vi "GUI_BELLA_ESP.vi"() -> ()   [LabVIEW 2013]
uses:
  Shared/GUI_Template/GUI_master/tcp_new_data_event.ctl
  Shared/GUI_Template/GUI_master/tcp new data cluster.ctl
panel:
  in  "stop":bool
  in  "Status.Axis 2::3":T1(ring) caption="Status"
  in  "Home.Axis 2::3":dbl=0.5 caption="Home" min=0.0 max=6.0 format="%_4f"
  in  "Power.Axis 2::3":enum16{"on", "off"}(ring) caption="Power"
  in  "Position.Axis 2::3":dbl=0.5 caption="Position" min=-12.0 max=10.0 format="%_4f"
  in  "Status.Axis 3::3":T1(ring) caption="Status"
  in  "Home.Axis 3::3":dbl=0.5 caption="Home" min=0.0 max=6.0 format="%_4f"
  in  "Power.Axis 3::3":enum16{"on", "off"}(ring) caption="Power"
  in  "Position.Axis 3::3":dbl=0.5 caption="Position" min=-12.0 max=12.0 format="%_4f"
  in  "Status.Axis 1::3":T1(ring) caption="Status"
  in  "Home.Axis 1::3":dbl=0.5 caption="Home" min=0.0 max=6.0 format="%_4f"
  in  "Power.Axis 1::3":enum16{"on", "off"}(ring) caption="Power"
  in  "Position.Axis 1::3":dbl=0.5 caption="Position" min=-10.0 max=10.0 format="%_4f"
  in  "Status.Axis 3::2":T1(ring) caption="Status"
  in  "Home.Axis 3::2":dbl=0.5 caption="Home" min=0.0 max=6.0 format="%_4f"
  in  "Power.Axis 3::2":enum16{"on", "off"}(ring) caption="Power"
  in  "Position.Axis 3::2":dbl=0.5 caption="Position" min=-10.0 max=10.0 format="%_4f"
  in  "Status.Axis 2::2":T1(ring) caption="Status"
  in  "Home.Axis 2::2":dbl=0.5 caption="Home" min=0.0 max=6.0 format="%_4f"
  in  "Power.Axis 2::2":enum16{"on", "off"}(ring) caption="Power"
  in  "Position.Axis 2::2":dbl=0.5 caption="Position" min=-6.0 max=3.0 format="%_4f"
  in  "Status.Axis 1::2":T1(ring) caption="Status"
  in  "Home.Axis 1::2":dbl=0.5 caption="Home" min=0.0 max=6.0 format="%_4f"
  in  "Power.Axis 1::2":enum16{"on", "off"}(ring) caption="Power"
  in  "Position.Axis 1::2":dbl=0.5 caption="Position" min=-8.0 max=3.0 format="%_4f"
  in  "Status.Axis 2::1":T1(ring) caption="Status"
  in  "Home.Axis 2::1":dbl=0.5 caption="Home" min=0.0 max=6.0 format="%_4f"
  in  "Power.Axis 2::1":enum16{"on", "off"}(ring) caption="Power"
  in  "Position.Axis 2::1":dbl=0.5 caption="Position" min=-3.0 max=3.0 format="%_4f"
  in  "Status.Axis 1::1":T1(ring) caption="Status"
  in  "Home.Axis 1::1":dbl=0.5 caption="Home" min=0.0 max=6.0 format="%_4f"
  in  "Power.Axis 1::1":enum16{"on", "off"}(ring) caption="Power"
  in  "Position.Axis 1::1":dbl=0.5 caption="Position" min=-10.0 max=10.0 format="%_4f"
  out "error IO 2":errorcluster
  out "tcp data event":T2
  in  "GUIdevice 3":string="BELLA_ESP_2"
  in  "GUIdevice 1":string="BELLA_ESP_M1"
  in  "GUIdevice 2":string="BellaESP"
  in  "insert tag":bool=TRUE
  # "Horizontal"
  # "BELLA PW ESP301"
  # "M5 AXIS 1"
  # "Horizontal"
  # "M5 AXIS 2"
  # "Vertical"
  # "M4 AXIS 2"
  # "Horizontal"
  # "M4 AXIS 1"
  # "Vertical"
  # "M2 AXIS 2"
  # "Horizontal"
  # "M2 AXIS 1"
  # "Vertical"
  # "M1 AXIS 2"
  # "Horizontal"
  # "M1 AXIS 1"
  # "Vertical"
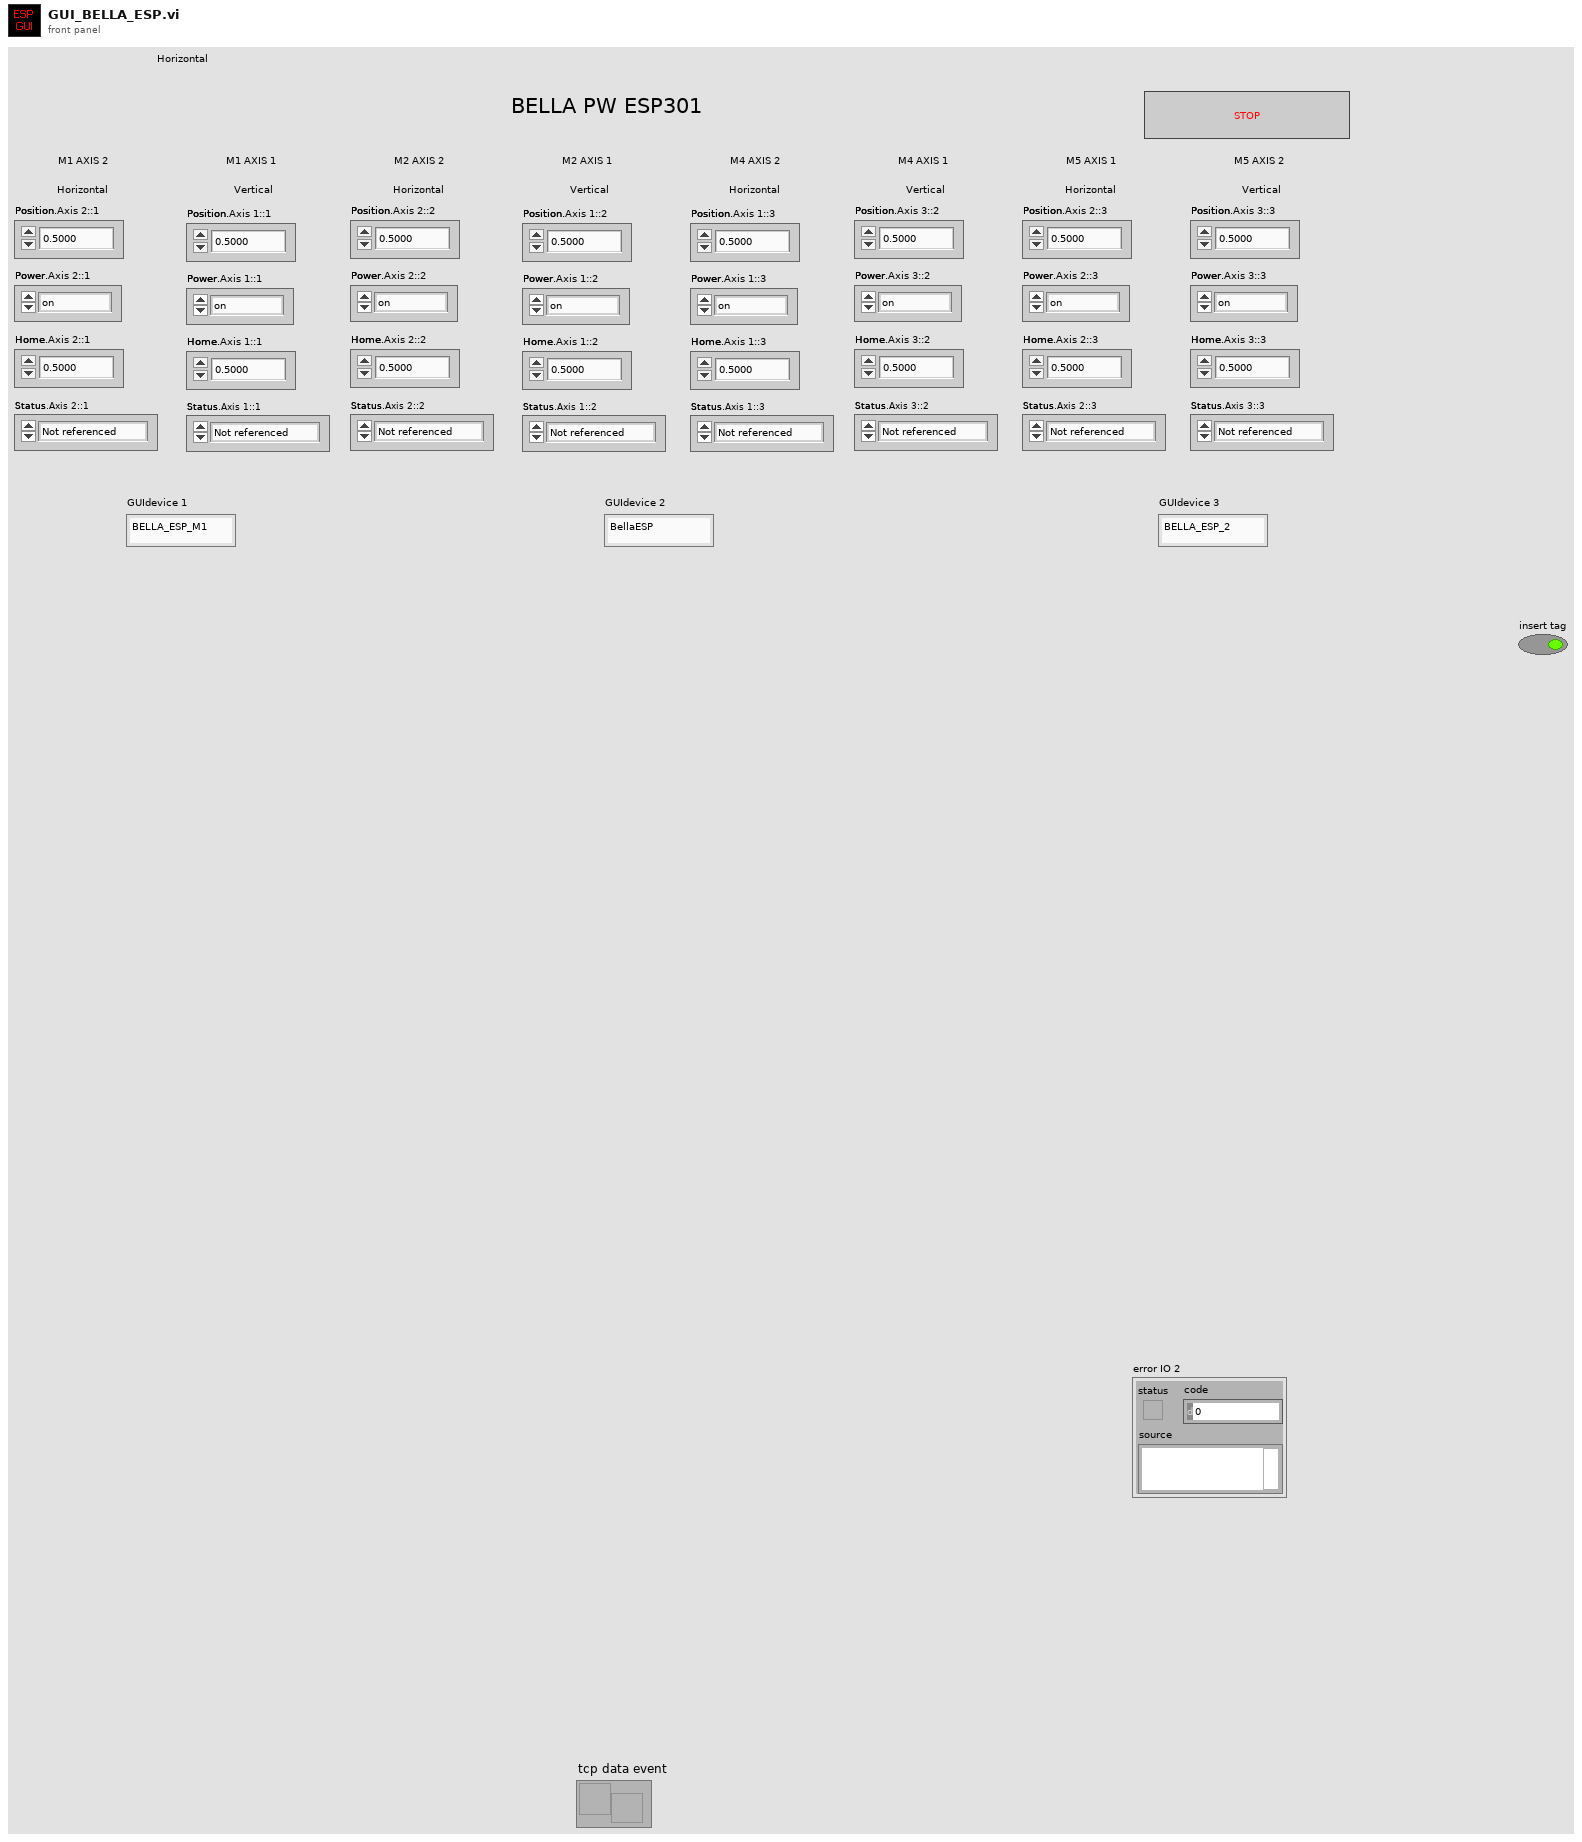
[diagram p1: front panel]
types:
  T1 = enum16{"Not referenced", "Homing", "Moving", "Ready"}
  T2 = typedef "tcp_new_data_event.ctl" = refnum<user-event>
  T3 = typedef "tcp new data cluster.ctl" = cluster{"EventEnum":enum16{"new data", "connection status update"}, "Device name":string}
  T4 = enum32{"Invalid", "Standard", "Closed", "Hidden", "Minimized", "Maximized"}
  T5 = enum32{"invalid app kind", "Development System", "Run Time System", "Student Edition", "Embedded LabVIEW", "Evaluation", "Custom"}
  T6 = cluster{"Core":cluster{"Current VI Reference":refnum<vi>, "Close Panel on Exit?":bool}, "Your Boolean data":bool, "Your string data":string}
  T7 = cluster{"Current VI Reference":refnum<vi>, "Close Panel on Exit?":bool}
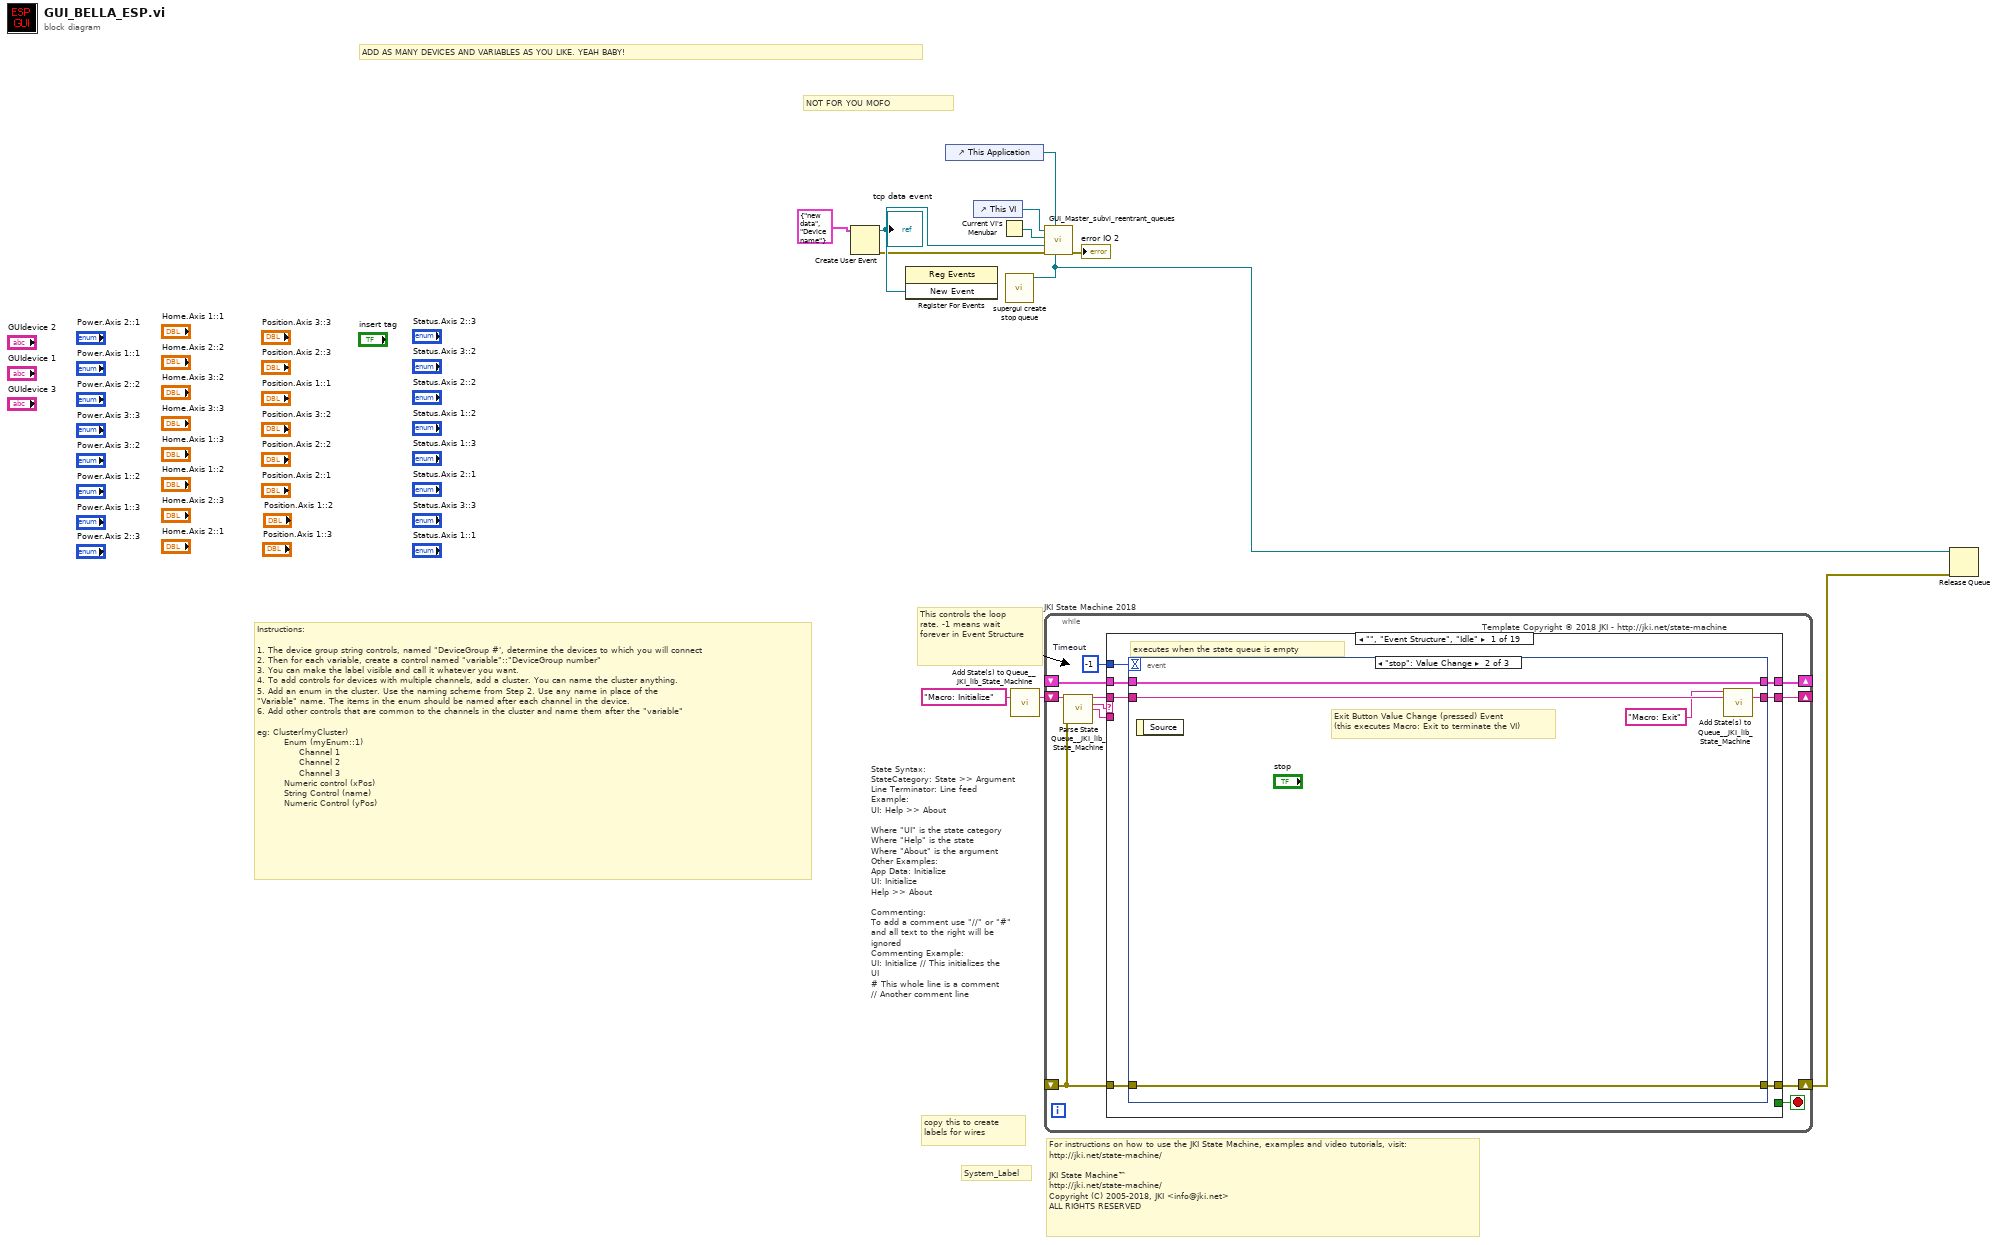
[diagram p0: block diagram]
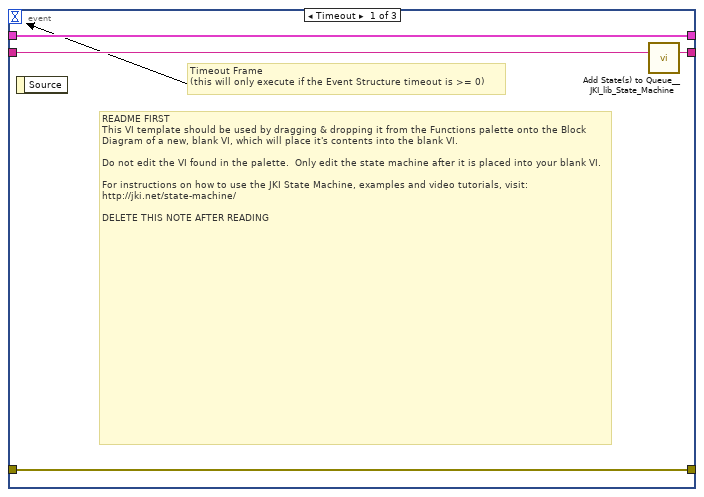
[diagram p2: hidden frame]
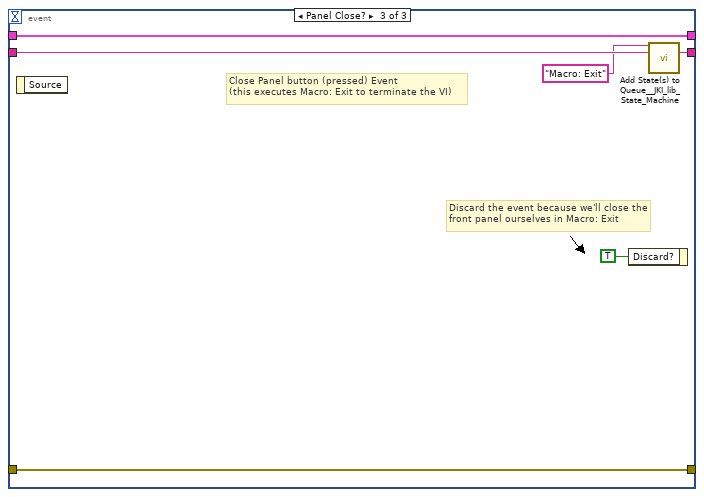
[diagram p3: hidden frame]
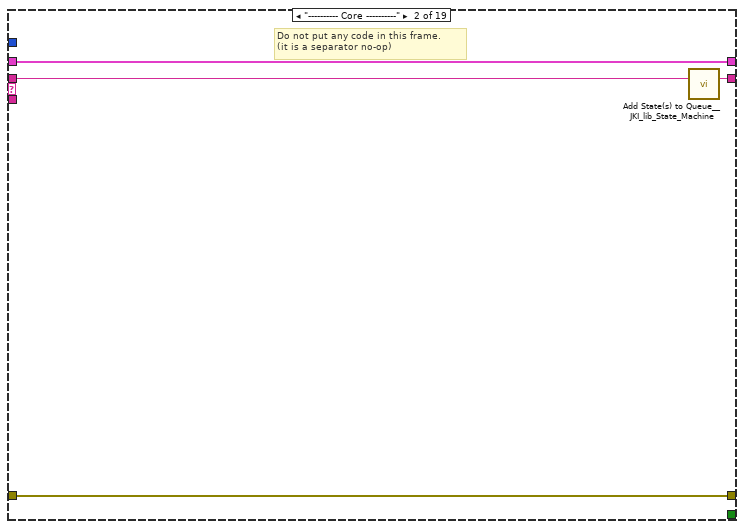
[diagram p4: hidden frame]
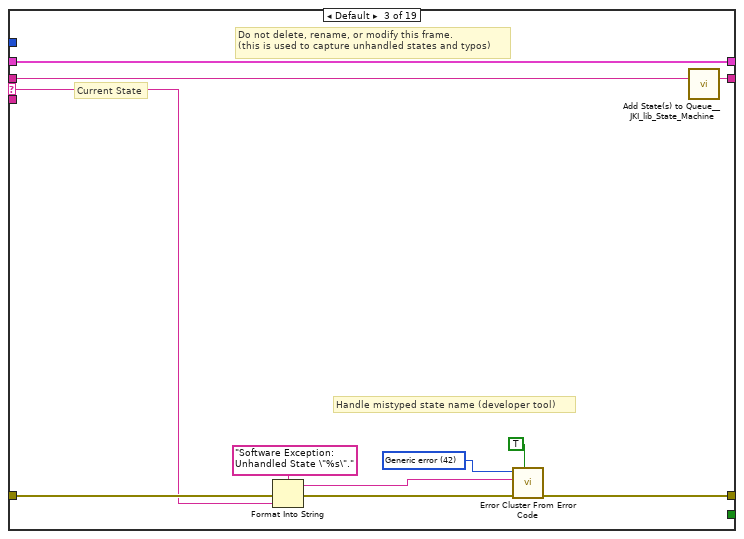
[diagram p5: hidden frame]
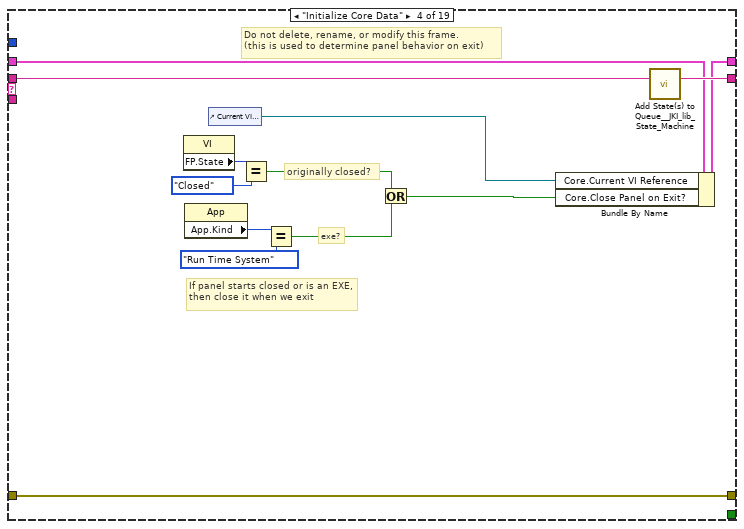
[diagram p6: hidden frame]
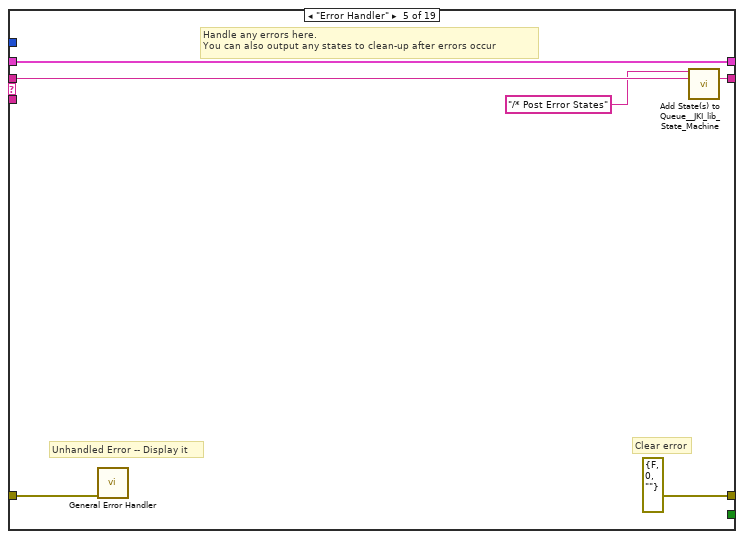
[diagram p7: hidden frame]
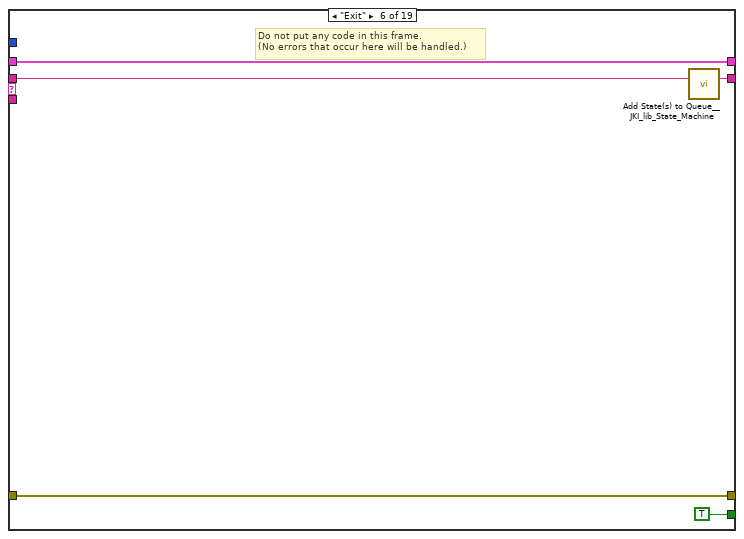
[diagram p8: hidden frame]
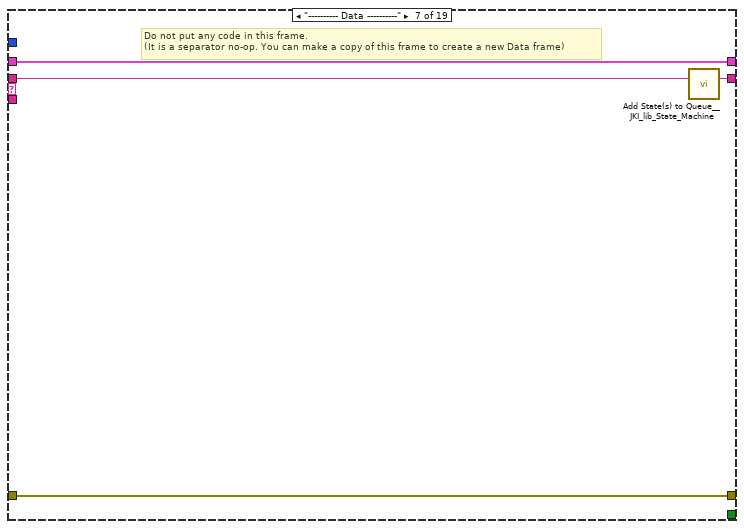
[diagram p9: hidden frame]
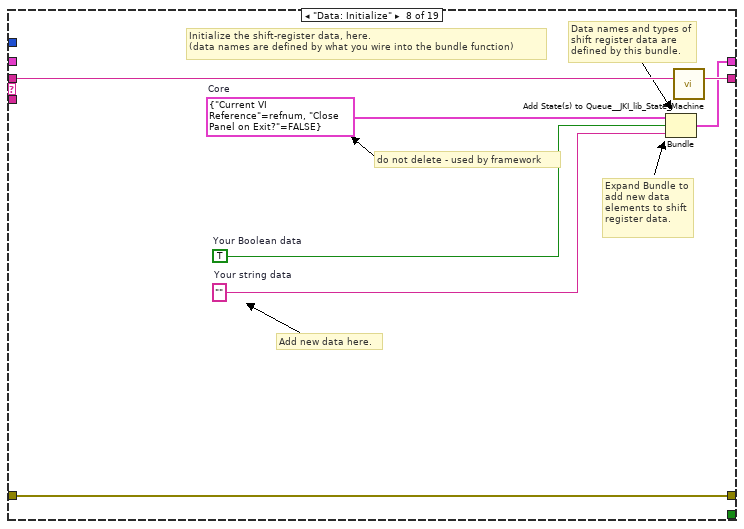
[diagram p10: hidden frame]
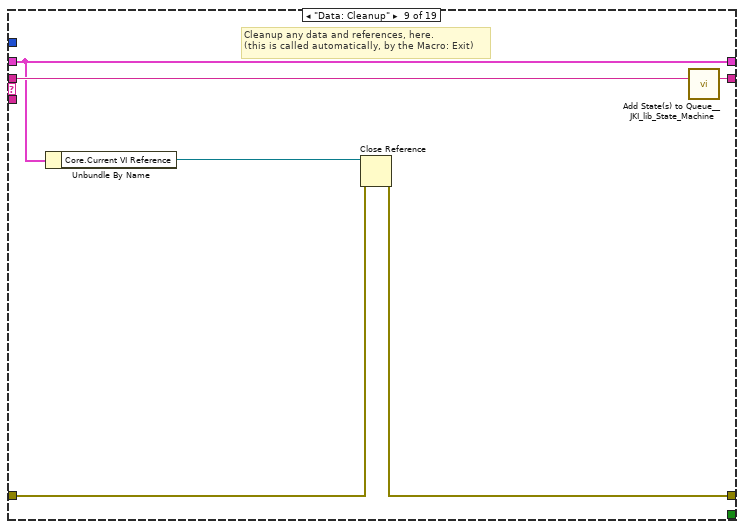
[diagram p11: hidden frame]
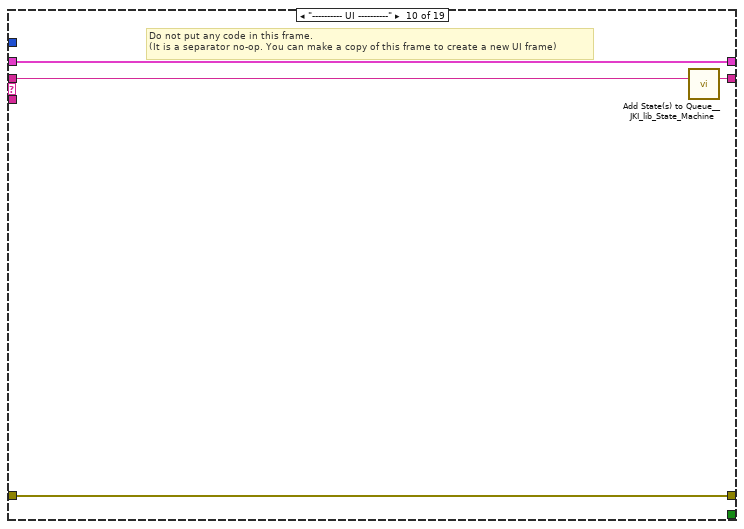
[diagram p12: hidden frame]
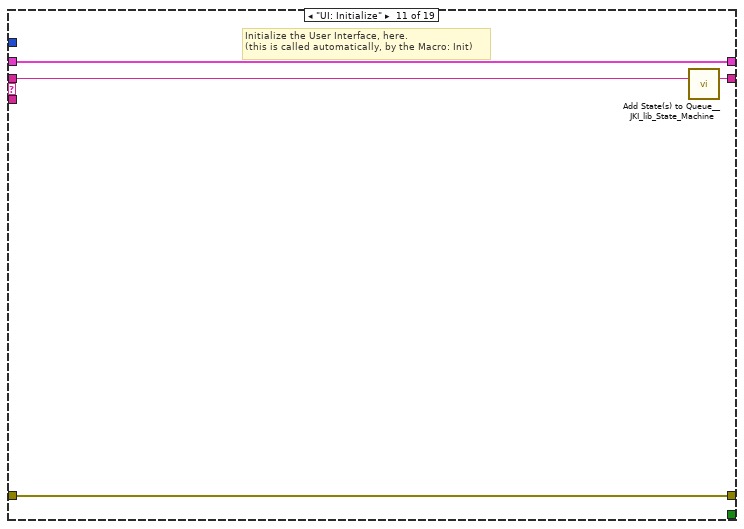
[diagram p13: hidden frame]
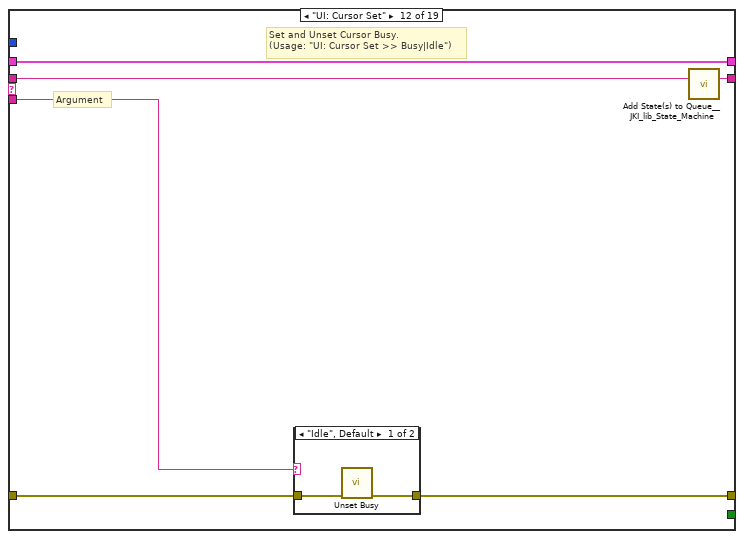
[diagram p14: hidden frame]
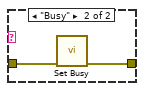
[diagram p15: hidden frame]
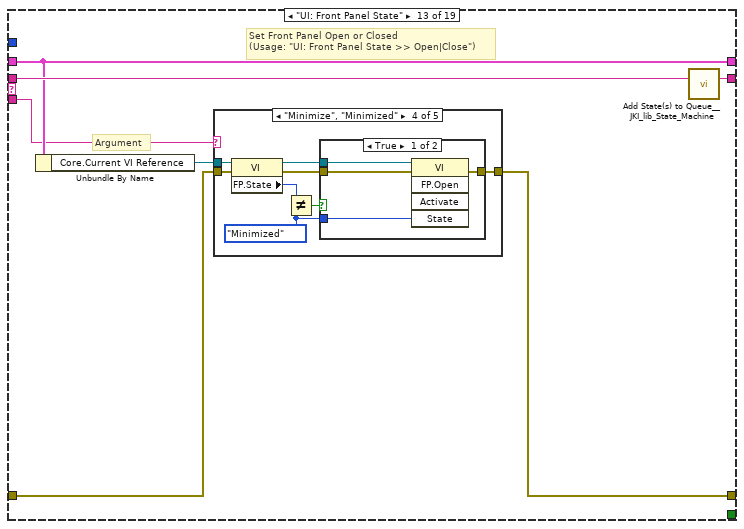
[diagram p16: hidden frame]
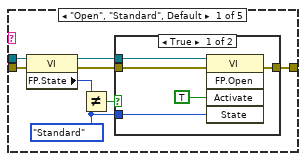
[diagram p17: hidden frame]
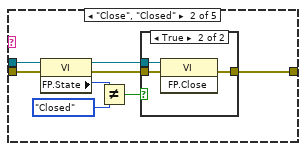
[diagram p19: hidden frame]
diagram:
  # "For instructions on how to use the JKI State Machine, examples and video tutorials, visit:\nhttp://jki.net/state-machine/\n\nJKI State Machine™\nhttp://jki.net/state-machine/\nCopyright (C) 2005-2018, JKI <info@jki.net>\nALL RIGHTS RESERVED"
  # "State Syntax:\nStateCategory: State >> Argument\nLine Terminator: Line feed\nExample:\nUI: Help >> About\n\nWhere \"UI\" is the state category\nWhere \"Help\" is the state\nWhere \"About\" is the argument\nOther Examples:\nApp Data: Initialize\nUI: Initialize\nHelp >> About\n\nCommenting:\nTo add a comment use \"//\" or \"#\" and all text to the right will be ignored\nCommenting Example:\nUI: Initialize // This initializes the UI\n# This whole line is a comment\n// Another comment line"
  # "copy this to create labels for wires"
  # "This controls the loop rate. -1 means wait forever in Event Structure"
  # "System_Label"
  # "NOT FOR YOU MOFO"
  # "Instructions:\n\n1. The device group string controls, named \"DeviceGroup #', determine the devices to which you will connect\n2. Then for each variable, create a control named \"variable\"::\"DeviceGroup number\"\n3. You can make the label visible and call it whatever you want.\n4. To add controls for devices with multiple channels, add a cluster. You can name the cluster anything.\n5. Add an enum in the cluster. Use the naming scheme from Step 2. Use any name in place of the \n\"Variable\" name. The items in the enum should be named after each channel in the device. \n6. Add other controls that are common to the channels in the cluster and name them after the \"variable\"\n\neg: Cluster(myCluster)\n         Enum (myEnum::1)\n              Channel 1 \n              Channel 2\n              Channel 3\n         Numeric control (xPos)\n         String Control (name)\n         Numeric Control (yPos)"
  # "ADD AS MANY DEVICES AND VARIABLES AS YOU LIKE. YEAH BABY!"
  n1 = Create User Event(user event datatype=T3 {"EventEnum"=enum."new data", "Device name"="Device name"} ("New Event")) -> (user event=w10:refnum<user-event>, error out=w9:errorcluster)  [unwired: 1 in]
  "tcp data event" <- w10
  n2 = register-events(w10) -> ()  [unwired: 2 in, 2 out]
  n3 = control-ref of="This Application"() -> (w11:refnum<vi>)
  n4 = control-ref of="This VI"() -> (w6:refnum<vi>)
  n5 = Current VI's Menubar() -> (w7:refnum<k9>)
  n6 = call "supergui create stop queue.vi"() -> ("STOP Queue out"=w4:refnum<queue>)  [unwired: 11 in]
  n7 = call <vilib>:"Add State(s) to Queue__JKI_lib_State_Machine.vi"("State(s) in (\"\")"="Macro: Initialize") -> ("States Out"=w3:string)  [unwired: 14 in]
  n8 = call "GUI_Master_subvi_reentrant_queues.vi"("STOP Queue in"=w4, "This Application"=w11, "error in (no error)"=w9, "tcp data event"=w10, "Caller menu reference"=w7, "Caller VI ref"=w6) -> ("error out"=→"error IO 2":errorcluster)  [unwired: 5 in]
  n9 = while "JKI State Machine 2018" {
    shift-right: [w15] -> _
    shift-left: _ -> [w14]
    shift-right: [w18] -> w1
    shift-left: _ -> [w12]
    shift-right: [w17] -> _
    shift-left: w3 -> [w19]
    stop <- w16 stop-if-true
    w13 = -1  # Timeout
    # "Template Copyright © 2018 JKI - http://jki.net/state-machine"
    n10 = call <vilib>:"Parse State Queue__JKI_lib_State_Machine.vi"("State Queue"=w19, "Error In (no error)"=w12) -> ("Remaining States"=w21:string, "Current State"=w22:string, "Arguments"=w20:string)  [unwired: 11 in]
    n11 = case shown="\"\", \"Event Structure\", \"Idle\"" w22 {
      selector: w22 -> [_ _ w49 _ _ _ _ _ _ _ _ _ _ _ _ _ _ _ _]
      tunnel: w21 -> [w29 w48 w53 w72 w78 w83 w87 w94 w100 w104 w108 w114 w125 w194 w199 w209 w213 w217 w221]
      tunnel: w20 -> [_ _ _ _ _ _ _ _ _ _ _ w109 w119 _ _ _ _ _ _]
      tunnel: w14 -> [w27 w45 w51 w65 w75 w81 w84 _ w95 w101 w106 w112 w121 w191 w196 w206 w210 w214 w218]
      tunnel: [w26 w46 w55 w69 errorcluster {"status"=FALSE, "code"=0, "source"=""} ("error out") w80 w85 w91 w96 w102 w105 w110 w122 w192 w197 w207 w211 w215 w219] -> w18
      tunnel: w12 -> [w25 w46 w54 w69 w74 w80 w85 w91 w97 w102 w105 w111 w123 w192 w197 w207 w211 w215 w219]
      tunnel: [w28 w47 w52 w71 w77 w82 w86 w93 w99 w103 w107 w113 w124 w193 w198 w208 w212 w216 w220] -> w17
      tunnel: [_ _ _ _ _ TRUE _ _ _ _ _ _ _ _ _ _ _ _ _] -> w16
      tunnel: [w24 w45 w51 w70 w75 w81 w84 w92 w95 w101 w106 w112 w121 w191 w196 w206 w210 w214 w218] -> w15
      tunnel: w13 -> [w23 _ _ _ _ _ _ _ _ _ _ _ _ _ _ _ _ _ _]
      frame "", "Event Structure", "Idle" {
        # "executes when the state queue is empty"
        n12 = event shown="[1] \"stop\": Value Change" {
          selector: _ -> [_ _ _]
          dyn-events: _ -> [_ _ _]
          timeout: w23 -> [_ _ _]
          tunnel: w29 -> [w33 w38 w44]
          tunnel: [w32 w37 w43] -> w28
          tunnel: w27 -> [w30 w35 w41]
          tunnel: [w31 w36 w42] -> w26
          tunnel: w25 -> [w31 w36 w42]
          tunnel: [w30 w35 w41] -> w24
          event Timeout {
            # "README FIRST\nThis VI template should be used by dragging & dropping it from the Functions palette onto the Block Diagram of a new, blank VI, which will place it's contents into the blank VI.\n\nDo not edit the VI found in the palette.  Only edit the state machine after it is placed into your blank VI.\n\nFor instructions on how to use the JKI State Machine, examples and video tutorials, visit:\nhttp://jki.net/state-machine/\n\nDELETE THIS NOTE AFTER READING"
            # "Timeout Frame\n(this will only execute if the Event Structure timeout is >= 0)"
            n13 = event-data() -> ()  [unwired: 1 in, 1 out]
            n14 = call <vilib>:"Add State(s) to Queue__JKI_lib_State_Machine.vi"("State(s) in (\"\")"=w33) -> ("States Out"=w32:string)  [unwired: 14 in]
          }
          event "stop": Value Change {
            # "Exit Button Value Change (pressed) Event\n(this executes Macro: Exit to terminate the VI)"
            n15 = event-data() -> ()  [unwired: 1 in, 1 out]
            n16 = call <vilib>:"Add State(s) to Queue__JKI_lib_State_Machine.vi"("State(s) in Front (\"\")"="Macro: Exit", "State(s) in (\"\")"=w38) -> ("States Out"=w37:string)  [unwired: 13 in]
          }
          event Panel Close? {
            # "Discard the event because we'll close the front panel ourselves in Macro: Exit"
            # "Close Panel button (pressed) Event\n(this executes Macro: Exit to terminate the VI)"
            n17 = event-data() -> ()  [unwired: 1 in, 1 out]
            n18 = event-data("Discard?"=TRUE) -> ()  [unwired: 1 in, 1 out]
            n19 = call <vilib>:"Add State(s) to Queue__JKI_lib_State_Machine.vi"("State(s) in Front (\"\")"="Macro: Exit", "State(s) in (\"\")"=w44) -> ("States Out"=w43:string)  [unwired: 13 in]
          }
        }
      }
      frame "---------- Core ----------" {
        # "Do not put any code in this frame.\n(it is a separator no-op)"
        n20 = call <vilib>:"Add State(s) to Queue__JKI_lib_State_Machine.vi"("State(s) in (\"\")"=w48) -> ("States Out"=w47:string)  [unwired: 14 in]
      }
      frame Default {
        w58 = 42 items=["No error", "Argument error", "Memory is full", "Out of zone", "End of file", "File already open", "Generic file I/O error", "File not found", "File permission error", "Disk is full", "Duplicate path", "Too many files open", "System feature not enabled", "Resource file not found", "Cannot add resource", "Resource not found", "Image not found", "Image memory error", "Pen does not exist", "Config type invalid", "Config token not found", "Config parse error", "Config memory error", "Bad external code format", "Bad external code offset", "External code not present", "Null window", "Destroy window error", "Null menu", "Print aborted", "Bad print record", "Print driver error", "Windows error during printing", "Memory error during printing", "Print dialog error", "Generic print error", "Invalid device refnum", "Device not found", "Device parameter error", "Device unit error", "Cannot open device", "Device call aborted", "Generic error", "Cancelled by user", "Object ID too low", "Object ID too high", "Object not in heap", "Unknown heap", "Unknown object (invalid DefProc)", "Unknown object (DefProc not in table)", "Message out of range", "Invalid (null) method", "Unknown message", "Manager call not supported", "Bad address", "Network operation in progress", "Network operation timed out", "Connection is busy", "Network attribute not supported", "Network error", "Address in use", "System out of memory", "Connection aborted", "Connection refused", "Not connected", "Already connected", "Connection closed", "Initialization error (interapplication manager)", "Bad occurrence", "Wait on unbound occurrence handler", "Occurrence queue overflow", "Datalog type conflict", "Unused", "Unrecognized type (interapplication manager)", "Memory corrupt", "Failed to make temporary DLL", "Old CIN version", "Drag socket not found", "Failed to load drop-object", "Failed to register OLE object", "Failed to release OLE object", "Format specifier type mismatch", "Unknown format specifier", "Too few format specifiers", "Too many format specifiers", "Scan failed", "Newer CIN version", "Error converting to variant", "Runtime menu error", "Password tampered", "Variant attribute not found", "Incompatible variant data type", "Event data is not available", "Event Store is not present", "Occurrence is not found", "Event Queue is not created", "Event info is not available", "Refnum passed is NULL", "Error retrieving Class GUID", "Error retrieving CoClass GUID", "Error retrieving TypeLib GUID.", "Bad built application magic bytes.", "Specific driver is different from the specific driver associated with the Logical Name.", "There is no session opened to the class driver.", "Max Error", "MAX - Error with config objects", "MAX - Error loading configuration", "MAX - Group not supported"]
        # "Current State"
        # "Do not delete, rename, or modify this frame.\n(this is used to capture unhandled states and typos)"
        # "Handle mistyped state name (developer tool)"
        n21 = Format Into String(format string="Software Exception: Unhandled State \"%s\"." ("message"), error in=w54, w49) -> (resulting string=w57:string, error out=w56:errorcluster)  [unwired: 1 in]
        n22 = call <vilib>:"Error Cluster From Error Code.vi"("show call chain? (False)"=TRUE, "error in (no error)"=w56, "error message (\"\")"=w57, "error code (0)"=w58) -> ("error out"=w55:errorcluster)  [unwired: 5 in]
        n23 = call <vilib>:"Add State(s) to Queue__JKI_lib_State_Machine.vi"("State(s) in (\"\")"=w53) -> ("States Out"=w52:string)  [unwired: 14 in]
      }
      frame "Initialize Core Data" {
        # "Do not delete, rename, or modify this frame.\n(this is used to determine panel behavior on exit)"
        # "originally closed?"
        # "exe?"
        # "If panel starts closed or is an EXE, then close it when we exit"
        n24 = property class="VI"() -> ("FP.State"=w62:T4)  [unwired: 2 in, 2 out]
        n25 = property class="App"() -> ("App.Kind"=w68:T5)  [unwired: 2 in, 2 out]
        n26 = control-ref of="Current VI Reference"() -> (w63:refnum<vi>)
        n27 = Equal?(x=w62, y=T4."Closed" ("Front Panel Window:State")) -> (x = y?=w60:bool)
        n28 = Equal?(x=w68, y=T5."Run Time System" ("Application:Kind")) -> (x = y?=w66:bool)
        n29 = Or(x=w60, y=w66) -> (x .or. y?=w64:bool)
        n30 = Bundle By Name(cluster=w65, "Core.Current VI Reference"=w63, "Core.Close Panel on Exit?"=w64) -> (w70:T6)
        n31 = call <vilib>:"Add State(s) to Queue__JKI_lib_State_Machine.vi"("State(s) in (\"\")"=w72) -> ("States Out"=w71:string)  [unwired: 14 in]
      }
      frame "Error Handler" {
        # "Unhandled Error -- Display it"
        # "Handle any errors here.\nYou can also output any states to clean-up after errors occur"
        # "Clear error"
        n32 = call <vilib>:"General Error Handler.vi"("error in (no error)"=w74) -> ()  [unwired: 10 in, 5 out]
        n33 = call <vilib>:"Add State(s) to Queue__JKI_lib_State_Machine.vi"("State(s) in Front (\"\")"="/* Post Error States", "State(s) in (\"\")"=w78) -> ("States Out"=w77:string)  [unwired: 13 in]
      }
      frame "Exit" {
        # "Do not put any code in this frame.\n(No errors that occur here will be handled.)"
        n34 = call <vilib>:"Add State(s) to Queue__JKI_lib_State_Machine.vi"("State(s) in (\"\")"=w83) -> ("States Out"=w82:string)  [unwired: 14 in]
      }
      frame "---------- Data ----------" {
        # "Do not put any code in this frame.\n(It is a separator no-op. You can make a copy of this frame to create a new Data frame)"
        n35 = call <vilib>:"Add State(s) to Queue__JKI_lib_State_Machine.vi"("State(s) in (\"\")"=w87) -> ("States Out"=w86:string)  [unwired: 14 in]
      }
      frame "Data: Initialize" {
        w88 = T7 {"Current VI Reference"=refnum, "Close Panel on Exit?"=FALSE}  # Core
        w90 = TRUE  # Your Boolean data
        w89 = ""  # Your string data
        # "do not delete - used by framework"
        # "Expand Bundle to add new data elements to shift register data."
        # "Add new data here."
        # "Data names and types of shift register data are defined by this bundle."
        # "Initialize the shift-register data, here.\n(data names are defined by what you wire into the bundle function)"
        n36 = Bundle("Core"=w88, "Your Boolean data"=w90, "Your string data"=w89) -> (w92:T6)  [unwired: 1 in]
        n37 = call <vilib>:"Add State(s) to Queue__JKI_lib_State_Machine.vi"("State(s) in (\"\")"=w94) -> ("States Out"=w93:string)  [unwired: 14 in]
      }
      frame "Data: Cleanup" {
        # "Cleanup any data and references, here.\n(this is called automatically, by the Macro: Exit)"
        n38 = Unbundle By Name(w95) -> ("Core.Current VI Reference"=w98:refnum<vi>)
        n39 = Close Reference(reference=w98, error in (no error)=w97) -> (error out=w96:errorcluster)
        n40 = call <vilib>:"Add State(s) to Queue__JKI_lib_State_Machine.vi"("State(s) in (\"\")"=w100) -> ("States Out"=w99:string)  [unwired: 14 in]
      }
      frame "---------- UI ----------" {
        # "Do not put any code in this frame.\n(It is a separator no-op. You can make a copy of this frame to create a new UI frame)"
        n41 = call <vilib>:"Add State(s) to Queue__JKI_lib_State_Machine.vi"("State(s) in (\"\")"=w104) -> ("States Out"=w103:string)  [unwired: 14 in]
      }
      frame "UI: Initialize" {
        # "Initialize the User Interface, here.\n(this is called automatically, by the Macro: Init)"
        n42 = call <vilib>:"Add State(s) to Queue__JKI_lib_State_Machine.vi"("State(s) in (\"\")"=w108) -> ("States Out"=w107:string)  [unwired: 14 in]
      }
      frame "UI: Cursor Set" {
        # "Argument"
        # "Set and Unset Cursor Busy.\n(Usage: \"UI: Cursor Set >> Busy|Idle\")"
        n43 = case shown="\"Idle\", Default" w109 {
          tunnel: w111 -> [w116 w118]
          tunnel: [w115 w117] -> w110
          frame "Idle", Default {
            n44 = call <vilib>:"Unset Busy.vi"("error in (no error)"=w116) -> ("error out"=w115:errorcluster)  [unwired: 10 in]
          }
          frame "Busy" {
            n45 = call <vilib>:"Set Busy.vi"("error in (no error)"=w118) -> ("error out"=w117:errorcluster)  [unwired: 9 in, 1 out]
          }
        }
        n46 = call <vilib>:"Add State(s) to Queue__JKI_lib_State_Machine.vi"("State(s) in (\"\")"=w114) -> ("States Out"=w113:string)  [unwired: 14 in]
      }
      frame "UI: Front Panel State" {
        # "Argument"
        # "Set Front Panel Open or Closed\n(Usage: \"UI: Front Panel State >> Open|Close\")"
        n47 = Unbundle By Name(w121) -> ("Core.Current VI Reference"=w120:refnum<vi>)
        n48 = case shown="\"Minimize\", \"Minimized\"" w119 {
          tunnel: w123 -> [w131 w146 w157 w170 w183]
          tunnel: [w133 w147 w159 w172 w185] -> w122
          tunnel: w120 -> [w132 w144 w158 w171 w184]
          frame "Open", "Standard", Default {
            w126 = T4."Standard" ("State")
            n49 = property class="VI"(reference=w132, error in=w131) -> (reference out=w129:refnum<vi>, error out=w130:errorcluster, "FP.State"=w128:T4)
            n50 = Not Equal?(x=w128, y=w126) -> (x != y?=w127:bool)
            n51 = case shown="True" w127 {
              tunnel: [w137 w139] -> w133
              tunnel: w130 -> [w136 w139]
              tunnel: w129 -> [w135 _]
              tunnel: w126 -> [w134 _]
              frame True {
                n52 = invoke class="VI" method="FP.Open"(reference=w135, error in=w136, "Activate"=TRUE, "State"=w134) -> (error out=w137:errorcluster)  [unwired: 1 in, 4 out]
              }
              frame False {
              }
            }
          }
          frame "Close", "Closed" {
            n53 = property class="VI"(reference=w144, error in=w146) -> (reference out=w143:refnum<vi>, error out=w145:errorcluster, "FP.State"=w141:T4)
            n54 = Not Equal?(x=w141, y=T4."Closed" ("Front Panel Window:State")) -> (x != y?=w140:bool)
            n55 = case shown="True" w140 {
              tunnel: [w148 w151] -> w147
              tunnel: w145 -> [w148 w150]
              tunnel: w143 -> [_ w149]
              frame False {
              }
              frame True {
                n56 = invoke class="VI" method="FP.Close"(reference=w149, error in=w150) -> (error out=w151:errorcluster)  [unwired: 1 in, 2 out]
              }
            }
          }
          frame "Hidden", "Hide" {
            w152 = T4."Hidden" ("State")
            n57 = property class="VI"(reference=w158, error in=w157) -> (reference out=w155:refnum<vi>, error out=w156:errorcluster, "FP.State"=w154:T4)
            n58 = Not Equal?(x=w154, y=w152) -> (x != y?=w153:bool)
            n59 = case shown="True" w153 {
              tunnel: [w163 w164] -> w159
              tunnel: w156 -> [w162 w164]
              tunnel: w155 -> [w161 _]
              tunnel: w152 -> [w160 _]
              frame True {
                n60 = invoke class="VI" method="FP.Open"(reference=w161, error in=w162, "State"=w160) -> (error out=w163:errorcluster)  [unwired: 2 in, 4 out]
              }
              frame False {
              }
            }
          }
          frame "Minimize", "Minimized" {
            w165 = T4."Minimized" ("State")
            n61 = property class="VI"(reference=w171, error in=w170) -> (reference out=w168:refnum<vi>, error out=w169:errorcluster, "FP.State"=w167:T4)
            n62 = Not Equal?(x=w167, y=w165) -> (x != y?=w166:bool)
            n63 = case shown="True" w166 {
              tunnel: [w176 w177] -> w172
              tunnel: w169 -> [w175 w177]
              tunnel: w168 -> [w174 _]
              tunnel: w165 -> [w173 _]
              frame True {
                n64 = invoke class="VI" method="FP.Open"(reference=w174, error in=w175, "State"=w173) -> (error out=w176:errorcluster)  [unwired: 2 in, 4 out]
              }
              frame False {
              }
            }
          }
          frame "Maximize", "Maximized" {
            w178 = T4."Maximized" ("State")
            n65 = property class="VI"(reference=w184, error in=w183) -> (reference out=w181:refnum<vi>, error out=w182:errorcluster, "FP.State"=w180:T4)
            n66 = Not Equal?(x=w180, y=w178) -> (x != y?=w179:bool)
            n67 = case shown="True" w179 {
              tunnel: [w189 w190] -> w185
              tunnel: w182 -> [w188 w190]
              tunnel: w181 -> [w187 _]
              tunnel: w178 -> [w186 _]
              frame True {
                n68 = invoke class="VI" method="FP.Open"(reference=w187, error in=w188, "State"=w186) -> (error out=w189:errorcluster)  [unwired: 2 in, 4 out]
              }
              frame False {
              }
            }
          }
        }
        n69 = call <vilib>:"Add State(s) to Queue__JKI_lib_State_Machine.vi"("State(s) in (\"\")"=w125) -> ("States Out"=w124:string)  [unwired: 14 in]
      }
      frame "---------- Macro ----------" {
        # "Do not put any code in this frame.\n(It is a separator no-op. You can make a copy of this frame to create a new Macro frame)"
        n70 = call <vilib>:"Add State(s) to Queue__JKI_lib_State_Machine.vi"("State(s) in (\"\")"=w194) -> ("States Out"=w193:string)  [unwired: 14 in]
      }
      frame "Macro: Initialize" {
        w195 = "Data: Initialize\nInitialize Core Data\nUI: Initialize\nUI: Front Panel State >> Open"  # Data: Initialize Initialize Core Data UI: Initialize UI: Front Panel State >> Open
        # "Initialization Macro\n(This is called once, when the VI starts)"
        n71 = call <vilib>:"Add State(s) to Queue__JKI_lib_State_Machine.vi"("State(s) in Front (\"\")"=w195, "State(s) in (\"\")"=w199) -> ("States Out"=w198:string)  [unwired: 13 in]
      }
      frame "Macro: Exit" {
        # "Exit Macro\n(This is called once, when the VI exits)"
        n72 = Unbundle By Name(w206) -> ("Core.Close Panel on Exit?"=w205:bool)
        n73 = Select(t="UI: Front Panel State >> Close", s=w205, f="") -> (s? t:f=w202:string)
        n74 = call <vilib>:"Add State(s) to Queue__JKI_lib_State_Machine.vi"("State(s) in (\"\")"=w202, "State(s) at Back (\"\")"="Data: Cleanup\nExit") -> ("States Out"=w200:string)  [unwired: 13 in]
        n75 = call <vilib>:"Add State(s) to Queue__JKI_lib_State_Machine.vi"("State(s) in Front (\"\")"=w200, "State(s) in (\"\")"=w209) -> ("States Out"=w208:string)  [unwired: 13 in]
      }
      frame "---------- New Category ----------" {
        # "Template Separator\n(You can make a copy of, or modify, this frame)"
        n76 = call <vilib>:"Add State(s) to Queue__JKI_lib_State_Machine.vi"("State(s) in (\"\")"=w213) -> ("States Out"=w212:string)  [unwired: 14 in]
      }
      frame "New Category: 1" {
        # "Your code here.\n(You can make a copy of, or modify, this frame)"
        n77 = call <vilib>:"Add State(s) to Queue__JKI_lib_State_Machine.vi"("State(s) in (\"\")"=w217) -> ("States Out"=w216:string)  [unwired: 14 in]
      }
      frame "New Category: 2" {
        # "Your code here.\n(You can make a copy of, or modify, this frame)"
        n78 = call <vilib>:"Add State(s) to Queue__JKI_lib_State_Machine.vi"("State(s) in (\"\")"=w221) -> ("States Out"=w220:string)  [unwired: 14 in]
      }
    }
  }
  n79 = Release Queue(queue=w4, error in (no error)=w1) -> ()  [unwired: 1 in, 3 out]
